vi "loadM100Recipe.vi"() -> ()   [LabVIEW 2012]
uses:
  <vilib>/Utility/NIReport.llb/NI_report.lvclass
  <vilib>/addons/database/Connection.llb/DB Tools Open Connec (Path).vi
  <vilib>/Utility/NIReport.llb/Excel/NI_Excel.lvclass
  <vilib>/addons/database/NI_Database_API.lvlib
panel:
  out "appended path":path
  out "data":string[][](array[string])
  out "error out 4":errorcluster
  in  "Cluster":T1
  out "number":i32
  out "error out 3":errorcluster
  in  "start cell":string="a2"
  out "error out":errorcluster
  in  "template (empty)":path=path "O:/Monitor/Recipe/PTSE/Module_Recipe Mapping Table.xls"
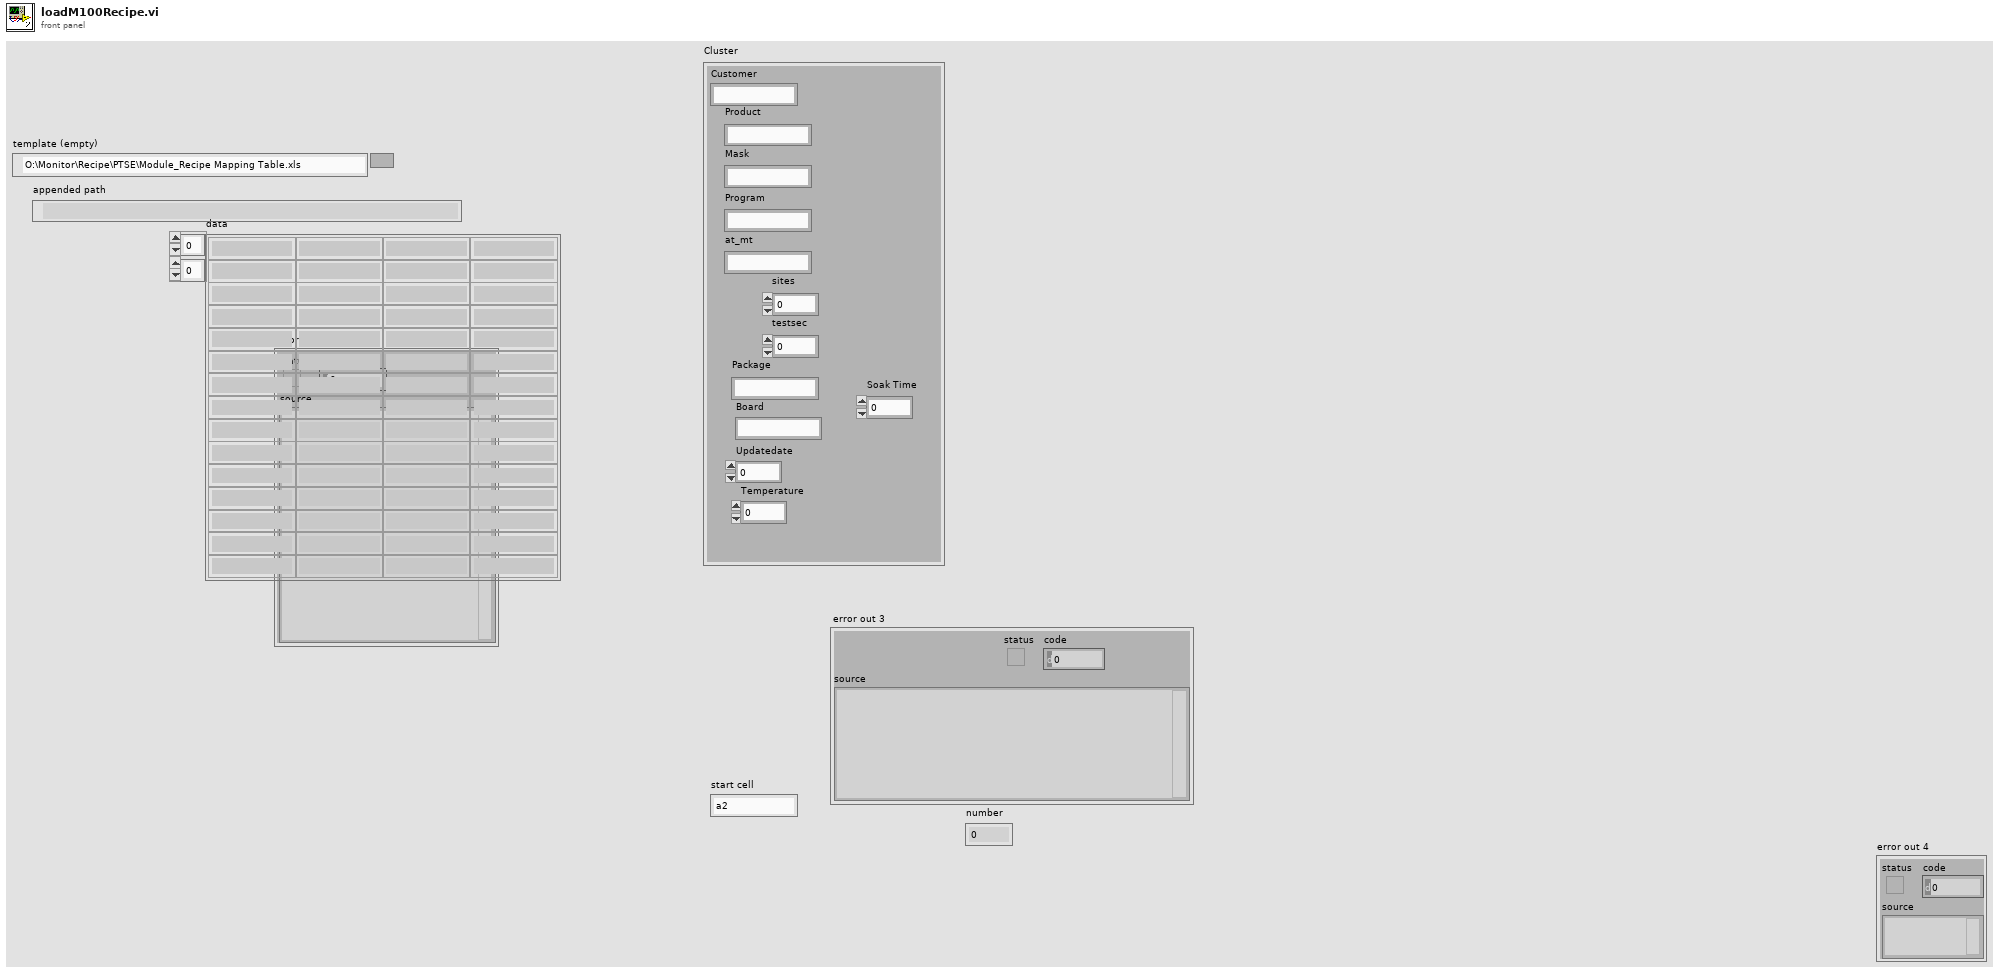
[diagram p1: front panel]
types:
  T1 = cluster{"Customer ":string, "Product":string, "Mask":string, "Program":string, "at_mt":string, "sites ":dbl, "testsec":dbl, "Package":string, "Board ":string, "Updatedate ":dbl, "Temperature":dbl, "Soak Time":dbl}
  T2 = enum16{"Standard Report", "HTML", "Word", "Excel"}
  T3 = typedef "NI_Database_API.lvlib/Conn ObjectReference.ctl" = refnum<k1>
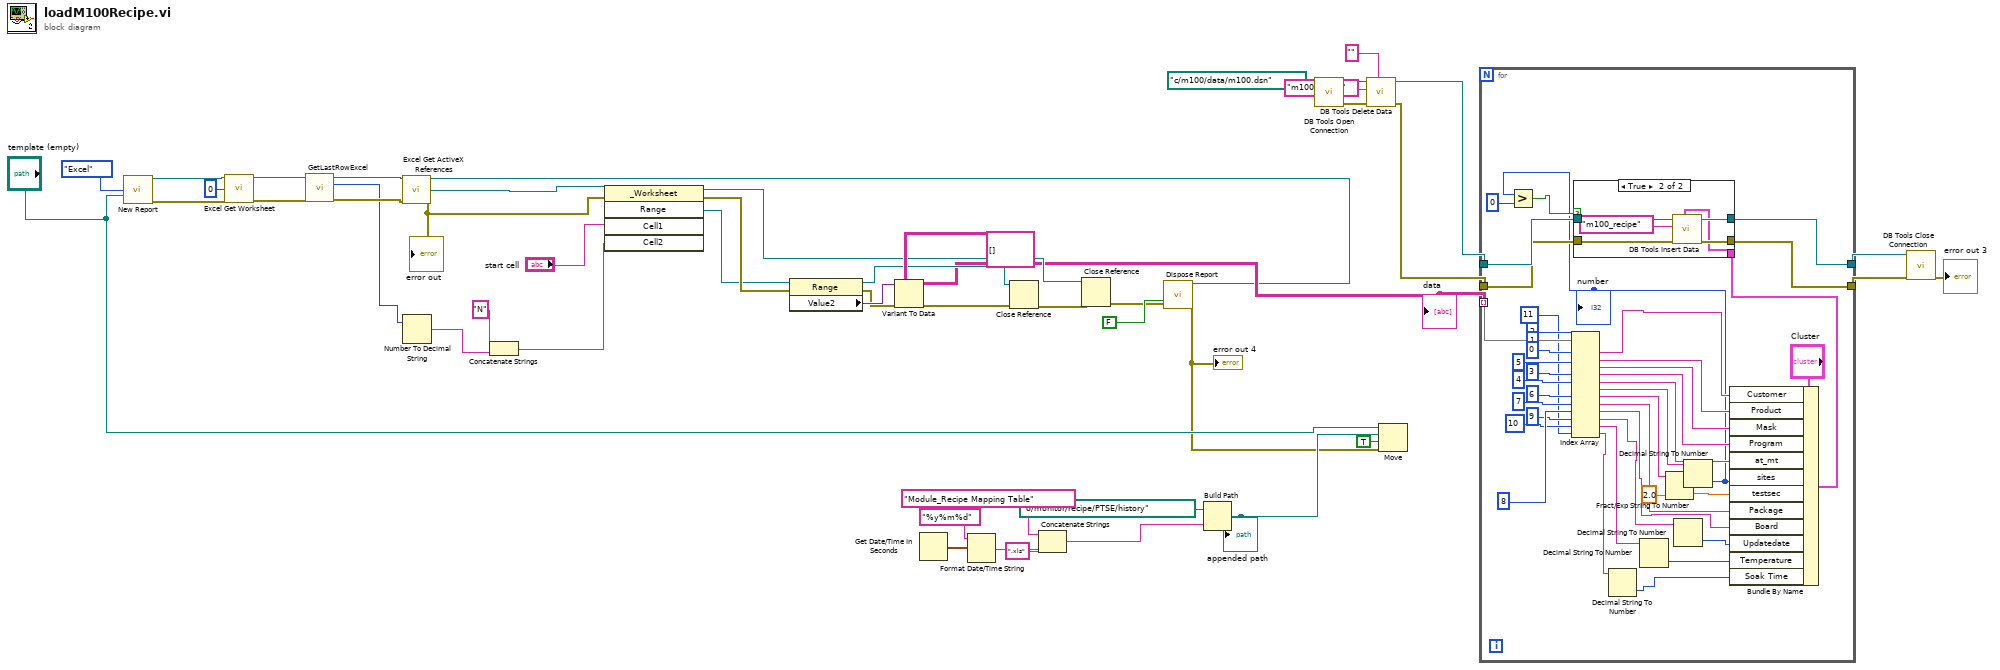
[diagram p0: block diagram]
diagram:
  n1 = call <vilib>:"New Report.vi"("report type"=T2."Excel", "template (empty)"="template (empty)") -> ("report out"=w48:refnum<class "NI_report.lvclass">, "error out"=w47:errorcluster)  [unwired: 12 in]
  n2 = call <vilib>:"Excel Get Worksheet.vi"("report in"=w48, "worksheet index (0)"=0, "error in (no error)"=w47) -> ("report out"=w28:refnum<class "NI_report.lvclass">, "error out"=w27:errorcluster)  [unwired: 11 in]
  n3 = call "GetLastRowExcel.vi"("error in (no error)"=w27, "report in"=w28) -> ("error out"=w25:errorcluster, "row"=w24:i32, "report out"=w26:refnum<class "NI_report.lvclass">)  [unwired: 7 in]
  n4 = call <vilib>:"Excel Get ActiveX References.vi"("report in"=w26, "error in (no error)"=w25) -> ("report out"=w18:refnum<class "NI_report.lvclass">, "Excel._Worksheet"=w44:refnum<k7>, "error out"=w29:errorcluster)  [unwired: 7 in, 4 out]
  "error out" <- w29
  n5 = Number To Decimal String(number=w24) -> (decimal integer string=w22:string)  [unwired: 1 in]
  n6 = Concatenate Strings("N" ("string"), w22) -> (w21:string)
  n7 = invoke class="_Worksheet" method="Range"(reference=w44, error in=w29, "Cell1"="start cell", "Cell2"=w21) -> (reference out=w36:refnum<k7>, error out=w41:errorcluster, "Range"=w40:refnum<k7>)  [unwired: 1 in, 2 out]
  n8 = property class="Range"(reference=w40, error in=w41) -> (reference out=w37:refnum<k7>, error out=w42:errorcluster, "Value2"=w43:variant)
  n9 = Variant To Data(error in=w42, type=string[][] [], Variant=w43) -> (data=w30:string[][], error out=w38:errorcluster)
  "data" <- w30
  n10 = Get Date/Time In Seconds() -> (seconds since 1Jan1904=w8:timestamp)
  n11 = Format Date/Time String(time format string (%c)="%y%m%d", seconds (now)=w8) -> (date/time string=w6:string)  [unwired: 1 in]
  n12 = Close Reference(reference=w37, error in (no error)=w38) -> (error out=w35:errorcluster)
  n13 = Concatenate Strings("Module_Recipe Mapping Table" ("string"), w6, ".xls" ("string")) -> (w9:string)
  n14 = Close Reference(reference=w36, error in (no error)=w35) -> (error out=w19:errorcluster)
  n15 = call-dynamic "Dispose Report.vi"("report in"=w18, "save changes? (F)"=FALSE, "error in (no error)"=w19) -> ("error out"=w2:errorcluster)  [unwired: 12 in]
  "error out 4" <- w2
  n16 = Build Path(base path=path "o:/monitor/recipe/PTSE/history", name or relative path=w9) -> (appended path=w3:path)
  "appended path" <- w3
  n17 = call-poly <vilib>:"DB Tools Open Connection.vi"("connection information"=path "c:/m100/data/m100.dsn") -> ("error out"=w17:errorcluster, "connection reference"=w16:T3)  [unwired: 7 in]
  n18 = call <vilib>:"DB Tools Delete Data.vi"("condition"="", "error in (no error)"=w17, "table"="m100_recipe", "connection reference"=w16) -> ("error out"=w14:errorcluster, "connection reference out"=w15:T3)  [unwired: 6 in]
  n19 = Move(source path="template (empty)", error in=w2, 9:TRUE ("overwrite (F)"), 10:w3) -> ()  [unwired: 1 in, 3 out]
  n20 = for {
    tunnel: w15 -> [w88]
    tunnel: w14 -> [w87]
    tunnel: [w86] -> w32
    tunnel: [w85] -> w31
    tunnel: w30 -> [w84] mode=indexing
    n21 = Index Array(array=w84, index #1=0 ("index"), index #2=1 ("index"), index #3=2 ("index"), index #4=3 ("index"), index #5=4 ("index"), index #6=5 ("index"), index #7=6 ("index"), index #8=7 ("index"), index #9=8 ("index"), index #10=9 ("index"), index #11=10 ("index"), index #12=11 ("index")) -> (element #1=w62:string, element #2=w70:string, element #3=w69:string, element #4=w68:string, element #5=w67:string, element #6=w58:string, element #7=w57:string, element #8=w66:string, element #9=w55:string, element #10=w54:string, element #11=w53:string, element #12=w52:string)
    n22 = Decimal String To Number(string=w52) -> (number=w61:i32)  [unwired: 2 in, 1 out]
    n23 = Decimal String To Number(string=w53) -> (number=w60:i32)  [unwired: 2 in, 1 out]
    n24 = Fract/Exp String To Number(string=w57, default (0 dbl)=2.0 ("default (0 DBL)")) -> (number=w56:dbl)  [unwired: 2 in, 1 out]
    n25 = Decimal String To Number(string=w54) -> (number=w59:i32)  [unwired: 2 in, 1 out]
    n26 = Decimal String To Number(string=w58) -> (number=w51:i32)  [unwired: 2 in, 1 out]
    "number" <- w51
    n27 = Greater?(x=w51, y=0) -> (0:w63:bool)
    n28 = Bundle By Name(cluster="Cluster", "Customer"=w62, "Product"=w70, "Mask"=w69, "Program"=w68, "at_mt"=w67, "sites"=w51, "testsec"=w56, "Package"=w66, "Board"=w55, "Updatedate"=w59, "Temperature"=w60, "Soak Time"=w61) -> (w65:T1)
    n29 = case shown="True" w63 {
      tunnel: w88 -> [w90 w95]
      tunnel: w87 -> [w89 w94]
      tunnel: [w90 w93] -> w86
      tunnel: [w89 w92] -> w85
      tunnel: w65 -> [_ w91]
      frame False {
      }
      frame True {
        n30 = call <vilib>:"DB Tools Insert Data.vi"("data"=w91, "error in (no error)"=w94, "table"="m100_recipe", "connection reference"=w95) -> ("error out"=w92:errorcluster, "connection reference out"=w93:T3)  [unwired: 6 in]
      }
    }
  }
  n31 = call <vilib>:"DB Tools Close Connection.vi"("error in (no error)"=w31, "connection reference"=w32) -> ("error out"=→"error out 3":errorcluster)  [unwired: 5 in]
